vi "Start Animation.vi"(8 "Error In":errorcluster, 11 "Animation Config":T1) -> (0 "Error Out":errorcluster, 3 "Animation Config":T1)   [LabVIEW 2011, in "LVH-Toolbox.lvlib" / "LVH-SystemTools.lvlib"]
uses:
  LVH-SystemTools.lvlib
  Private/UI/Animations/Animation Config.ctl
  <vilib>/picture/picture.llb/imagedata.ctl
  Private/UI/Type Defs/FGV States.ctl
panel:
  in  "Error In 2":errorcluster
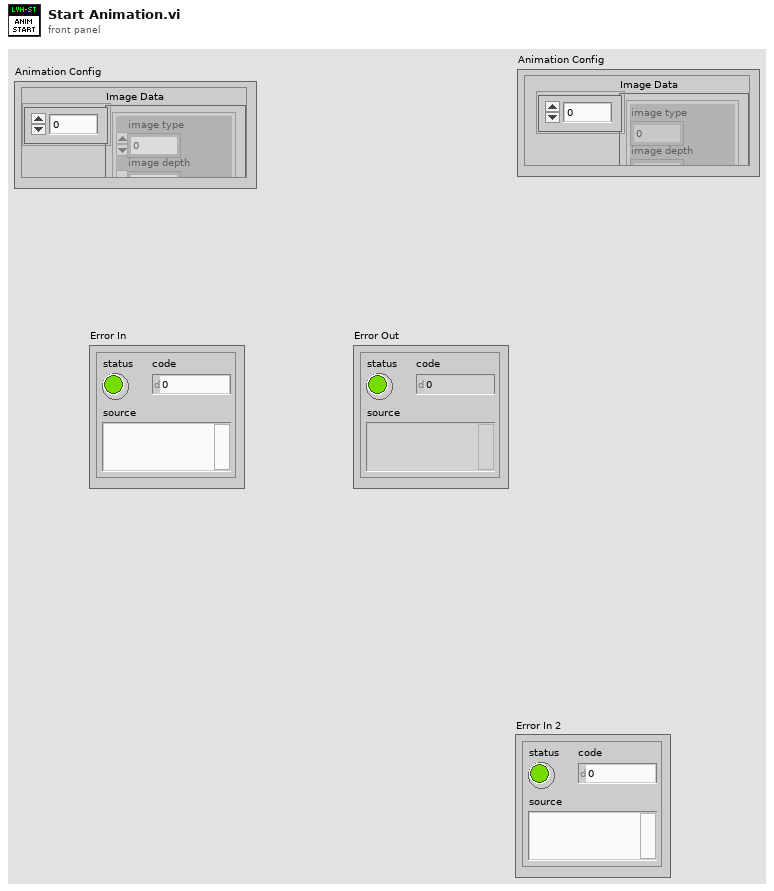
[diagram p1: front panel]
types:
  T1 = typedef "LVH-Toolbox.lvlib/LVH-SystemTools.lvlib/Animation Config.ctl" = cluster{"Image Data":T2[], "FPS":u32, "Position":cluster{"X":i16, "Y":i16}}
  T2 = typedef "imagedata.ctl" = cluster{"image type":i32, "image depth":i32, "image":u8[], "mask":u8[], "colors":u32[], "Rectangle":cluster{"left":i16, "top":i16, "right":i16, "bottom":i16}}
  T3 = enum32{"invalid app kind", "Development System", "Run Time System", "Student Edition", "Embedded LabVIEW", "Evaluation", "Custom"}
  T4 = typedef "LVH-Toolbox.lvlib/LVH-SystemTools.lvlib/FGV States.ctl" = enum16{"Init", "Set", "Get"}
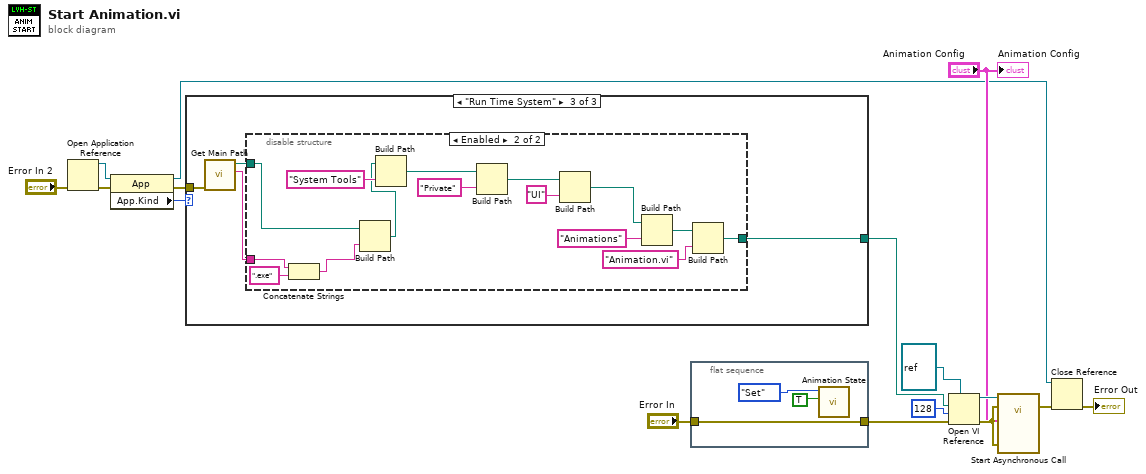
[diagram p0: block diagram]
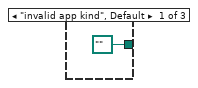
[diagram p2: hidden frame]
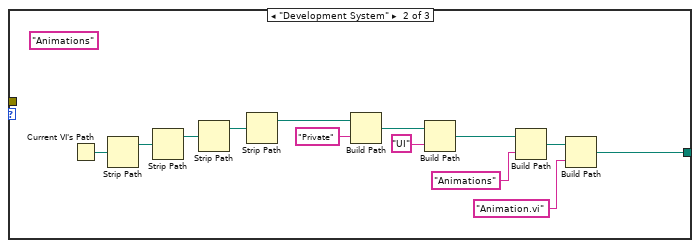
[diagram p3: hidden frame]
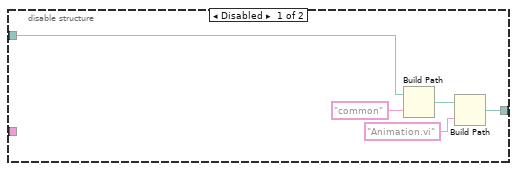
[diagram p4: hidden frame]
diagram:
  n1 = Open Application Reference(8:"Error In 2") -> (0:w8:errorcluster, 3:w7:refnum<vi>)  [unwired: 3 in]
  n2 = property class="App"(reference=w7, error in=w8) -> (reference out=w1:refnum<vi>, error out=w4:errorcluster, "App.Kind"=w6:T3)
  n3 = case shown="\"Run Time System\"" w6 {
    tunnel: [path "" ("appended path") w19 w32] -> w5
    tunnel: w4 -> [_ _ w33]
    frame "invalid app kind", Default {
    }
    frame "Development System" {
      (unwired) "Animations" ("name or relative path")
      n4 = Current VI's Path() -> (path=w28:path)
      n5 = Strip Path(path=w28) -> (stripped path=w23:path)  [unwired: 1 out]
      n6 = Strip Path(path=w23) -> (stripped path=w24:path)  [unwired: 1 out]
      n7 = Strip Path(path=w24) -> (stripped path=w29:path)  [unwired: 1 out]
      n8 = Strip Path(path=w29) -> (stripped path=w30:path)  [unwired: 1 out]
      n9 = Build Path(base path=w30, name or relative path="Private") -> (appended path=w25:path)
      n10 = Build Path(base path=w25, name or relative path="UI") -> (appended path=w26:path)
      n11 = Build Path(base path=w26, name or relative path="Animations") -> (appended path=w27:path)
      n12 = Build Path(base path=w27, name or relative path="Animation.vi") -> (appended path=w19:path)
    }
    frame "Run Time System" {
      n13 = call "Get Main Path.vi"("Error In"=w33) -> ("Main Name"=w31:string, "Main Dir"=w34:path)  [unwired: 8 in, 1 out]
      n14 = disable-structure shown="Enabled" {
        disable-tunnel: w34 -> [w39 w43]
        disable-tunnel: [w35 w49] -> w32
        disable-tunnel: w31 -> [_ w41]
        frame Disabled {
          n15 = Build Path(base path=w39, name or relative path="common") -> (appended path=w36:path)
          n16 = Build Path(base path=w36, name or relative path="Animation.vi") -> (appended path=w35:path)
        }
        frame Enabled {
          n17 = Concatenate Strings(w41, ".exe" ("string")) -> (w40:string)
          n18 = Build Path(base path=w43, name or relative path=w40) -> (appended path=w44:path)
          n19 = Build Path(base path=w44, name or relative path="System Tools") -> (appended path=w48:path)
          n20 = Build Path(base path=w48, name or relative path="Private") -> (appended path=w47:path)
          n21 = Build Path(base path=w47, name or relative path="UI") -> (appended path=w46:path)
          n22 = Build Path(base path=w46, name or relative path="Animations") -> (appended path=w45:path)
          n23 = Build Path(base path=w45, name or relative path="Animation.vi") -> (appended path=w49:path)
        }
      }
    }
  }
  n24 = flat-sequence {
    tunnel: [w55] -> w14
    tunnel: "Error In" -> [w55]
    frame #0 {
      n25 = call "Animation State.vi"("Running?"=TRUE, "Function"=FGV_States."Set") -> ()  [unwired: 9 in, 1 out]
    }
  }
  n26 = Open VI Reference(type specifier VI Refnum (for type only)=refnum<vi> refnum, vi path=w5, options=128, error in (no error)=w14) -> (vi reference=w11:refnum<vi>, error out=w13:errorcluster)  [unwired: 2 in]
  n27 = call-by-ref "Start Asynchronous Call"(reference=w11, error in=w13, "Error In"=w13, "Animation Config"="Animation Config") -> (error out=w3:errorcluster)  [unwired: 8 in, 3 out]
  n28 = Close Reference(reference=w1, error in (no error)=w3) -> (error out=→"Error Out":errorcluster)
  "Animation Config" <- "Animation Config"
